vi "Get Notebook ID.vi"(8 "Error In (No Error)":errorcluster, 9 "User":string="myemail", 10 "Notebook Name":string="My notebook on One Drive", 11 "client handle":T1) -> (0 "Error Out":errorcluster, 1 "key not found?":bool, 2 "Notebook ID":string, 3 "client handle out":T1, 4 "Header Value":string, 5 "body":string)   [LabVIEW 2019, in "OneNote Library.lvlib"]
uses:
  OneNote Library.lvlib
  <vilib>/httpClient/ClientHandle.ctl
  <vilib>/JDP Science/JSONtext/String Subset.vi
  <vilib>/JDP Science/JSONtext/support/Strip Quotes and Unescape.vi
  <vilib>/JDP Science/JSONtext/support/Unescape JSON string.vi
  <vilib>/JDP Science/JSONtext/Parsing/Parse Full Path or Item Name.vi
  <vilib>/JDP Science/JSONtext/Offset/Find Item Locations by Path.vi
  Useful OAuth VIs/globals.vi
  <vilib>/httpClient/LabVIEWHTTPClient.lvlib
  Useful OAuth VIs/Useful OAuth VIs.lvlib
  <vilib>/JDP Science/JSONtext/JSONtext.lvlib
  Useful HTTP VIs/Useful HTTP VIs.lvlib
panel:
  out "Output Header":string
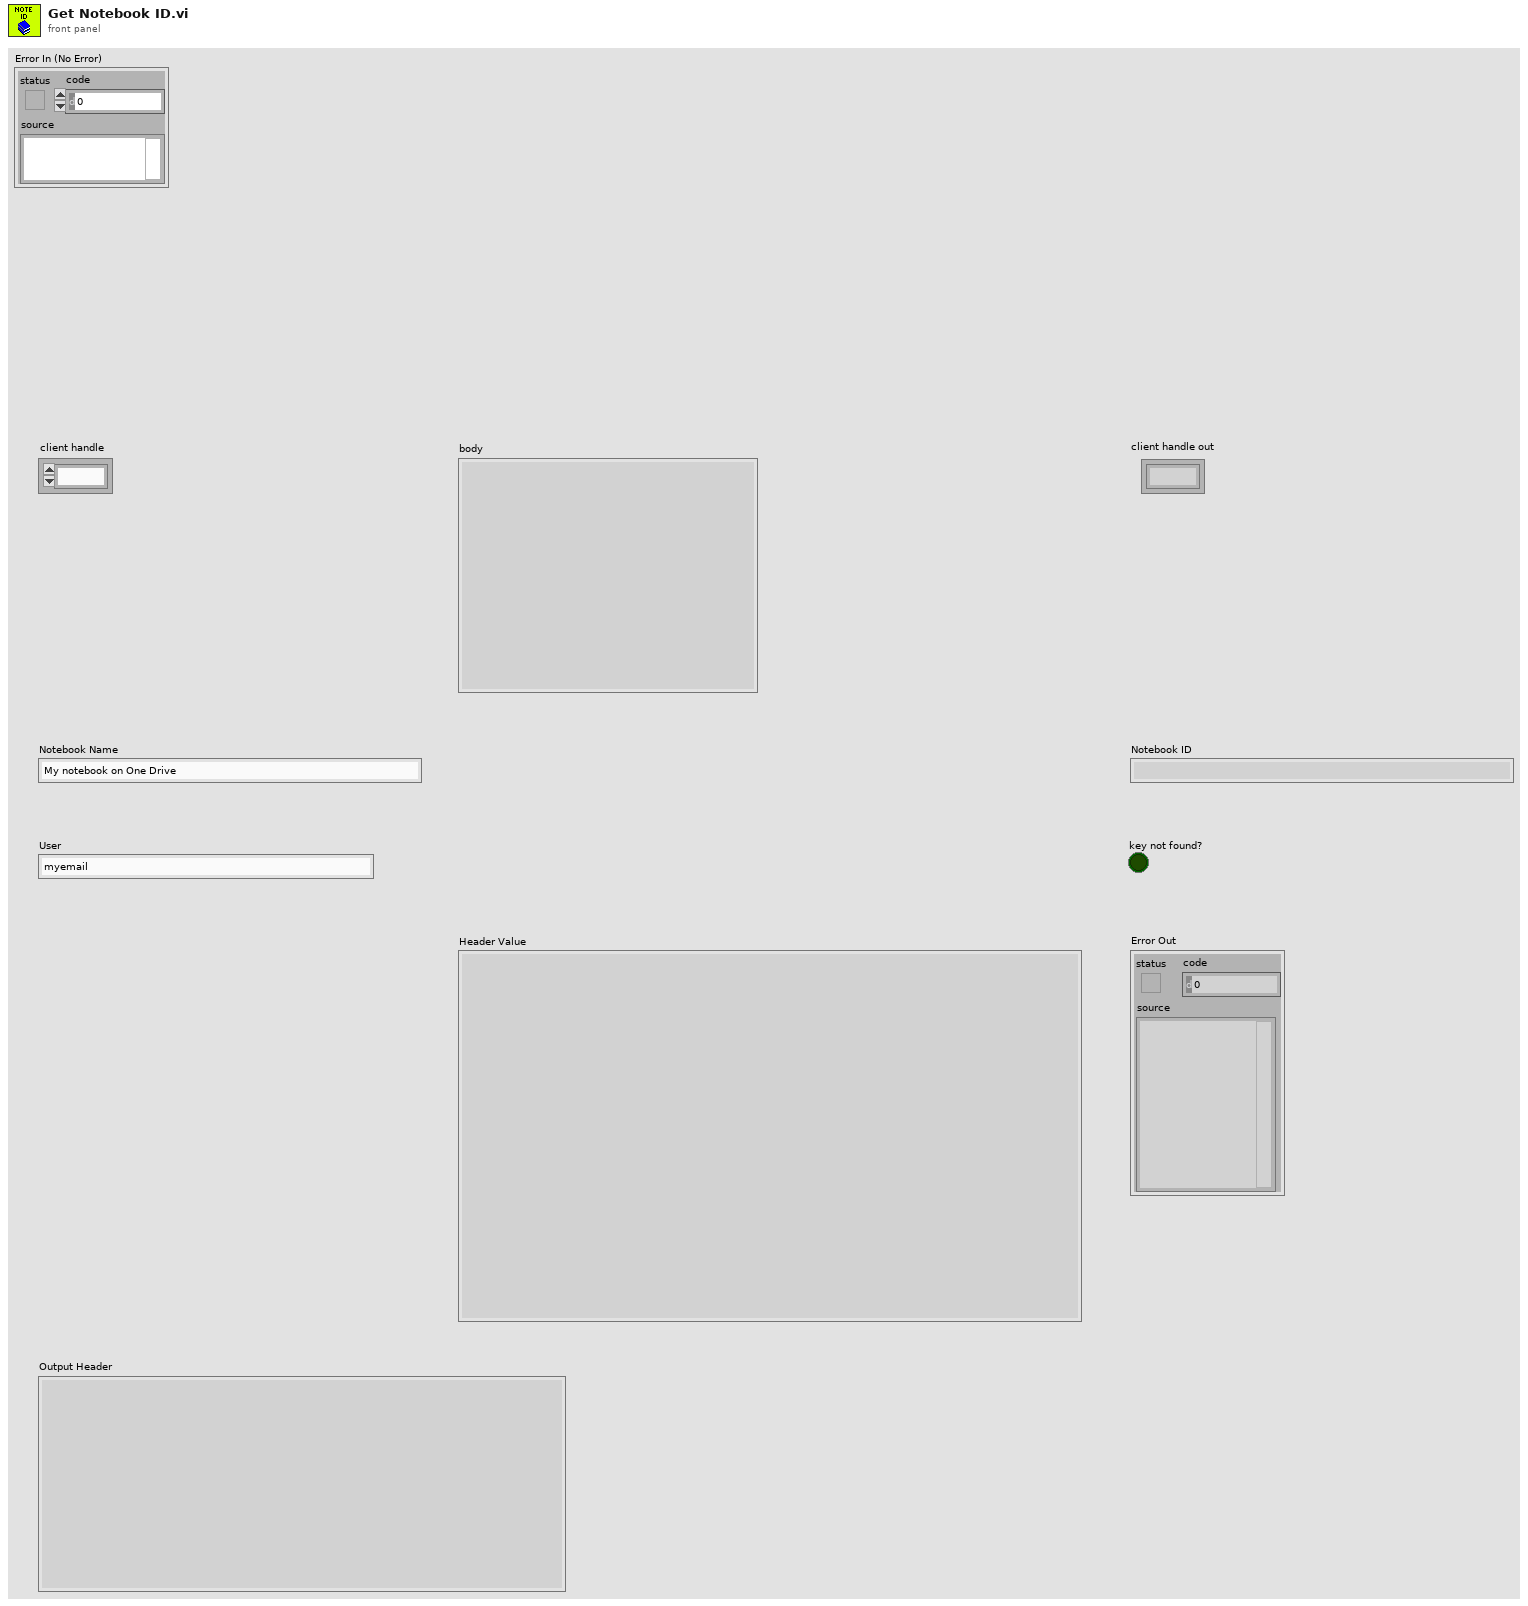
[diagram p1: front panel]
types:
  T1 = typedef "LabVIEWHTTPClient.lvlib/ClientHandle.ctl" = refnum<k1>
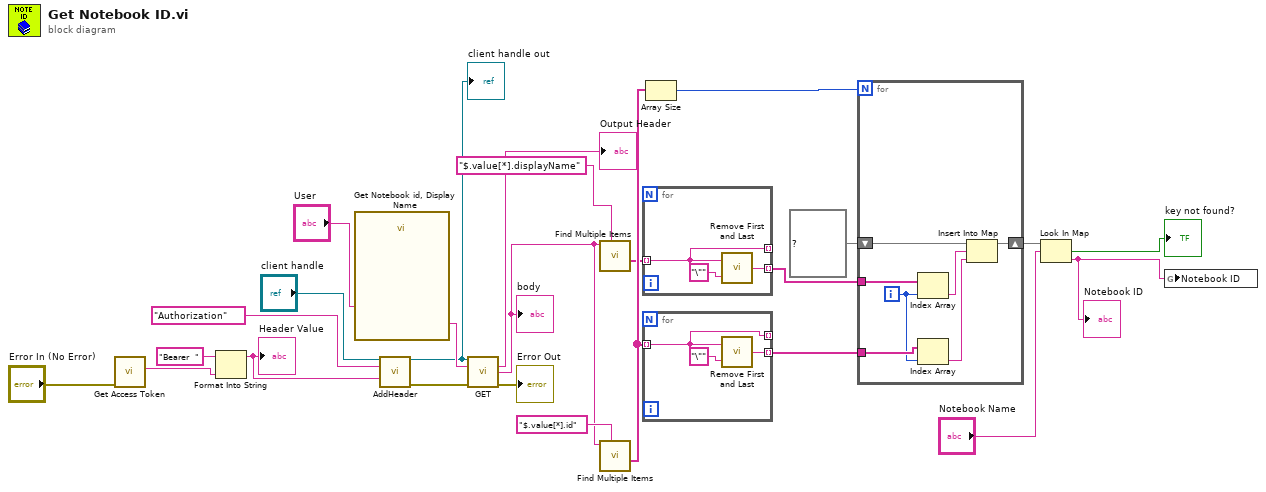
[diagram p0: block diagram]
diagram:
  n1 = call "Get Access Token.vi"("Error In (No Error)"="Error In (No Error)") -> ("access token"=w23:string)  [unwired: 9 in, 1 out]
  n2 = Format Into String(initial string="Bearer  ", w23) -> (resulting string=w22:string)  [unwired: 2 in, 1 out]
  "Header Value" <- w22
  n3 = call "Get Notebook id, Display Name"("user"="User") -> ("Result"=w18:string)  [unwired: 13 in, 1 out]
  n4 = call <vilib>:"AddHeader.vi"("client handle"="client handle", "header"="Authorization", "value"=w22) -> ("client handle out"=w4:T1, "error out"=w21:errorcluster)  [unwired: 11 in]
  "client handle out" <- w4
  n5 = call <vilib>:"GET.vi"("client handle"=w4, "url"=w18, "error in (no error)"=w21) -> ("headers"=→"Output Header":string, "body"=w6:string, "error out"=→"Error Out":errorcluster)  [unwired: 9 in, 1 out]
  "body" <- w6
  n6 = call <vilib>:"Find Multiple Items.vi"("$Path or Item Name"="$.value[*].displayName", "JSON"=w6) -> ("<JSON>"=w14:string[])  [unwired: 6 in, 3 out]
  n7 = call <vilib>:"Find Multiple Items.vi"("$Path or Item Name"="$.value[*].id", "JSON"=w6) -> ("<JSON>"=w16:string[])  [unwired: 6 in, 3 out]
  n8 = for {
    tunnel: w14 -> [w26] mode=indexing
    tunnel: [w26] -> _ mode=indexing
    tunnel: [w27] -> w11 mode=indexing
    n9 = call "Remove First and Last.vi"("Char to Remove"="\"", "String"=w26) -> ("Result"=w27:string)
  }
  n10 = for {
    tunnel: w16 -> [w29] mode=indexing
    tunnel: [w29] -> _ mode=indexing
    tunnel: [w30] -> w13 mode=indexing
    n11 = call "Remove First and Last.vi"("Char to Remove"="\"", "String"=w29) -> ("Result"=w30:string)
  }
  n12 = Array Size(array=w16) -> (size(s)=w12:i32)
  n13 = for {
    N: w12 -> [_]
    tunnel: w13 -> [w38]
    tunnel: w11 -> [w37]
    shift-right: [w34] -> w9
    shift-left: map{string, string} {} ("map") -> [w36]
    i -> [w35]
    n14 = Index Array(array=w37, index=w35) -> (element=w33:string)
    n15 = Index Array(array=w38, index=w35) -> (element=w32:string)
    n16 = Insert Into Map(map in=w36, key=w33, value=w32) -> (map out=w34:map{string, string})  [unwired: 2 out]
  }
  n17 = Look In Map(map=w9, key="Notebook Name") -> (key not found?=→"key not found?":bool, value=w2:string)  [unwired: 1 in]
  "Notebook ID" <- w2
  n18 = global write "globals.vi" "Notebook ID"(w2) -> ()
